vi "generateOriGrating.vi"(0 "Y resolution":i32=128, 1 "Square?":bool, 2 "New Image":T1, 5 "X resolution":i32, 7 "frequency (cyc/pixel)":dbl=0.0078125 format="%0.4e", 9 "Angle (degrees)":sgl format="%.2f", 11 "error in (no error)":errorcluster, 12 "phase in":dbl format="%0.2f") -> (4 "Image Dst Out":T1, 15 "error out":errorcluster)   [LabVIEW 2014]
uses:
  <vilib>/vision/Image Controls.llb/IMAQ Image.ctl
  <vilib>/Analysis/baseanly.llb/Real Outer Product.vi
  <vilib>/Analysis/Matrix/Numeric/Multiply/Multiply - RM,R.vi
  <vilib>/Analysis/NI_AALBase.lvlib
  <vilib>/Analysis/Matrix/NI_Matrix.lvlib
  <vilib>/vision/NI_Vision_Development_Module.lvlib
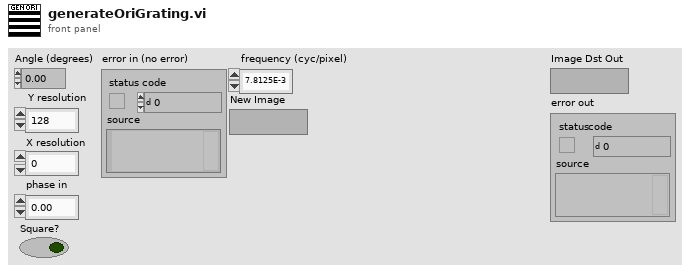
[diagram p1: front panel]
types:
  T1 = typedef "IMAQ Image.ctl" = refnum<image>
  T2 = typedef "NI_Matrix.lvlib/RealMatrix.ctl" = dbl[][]
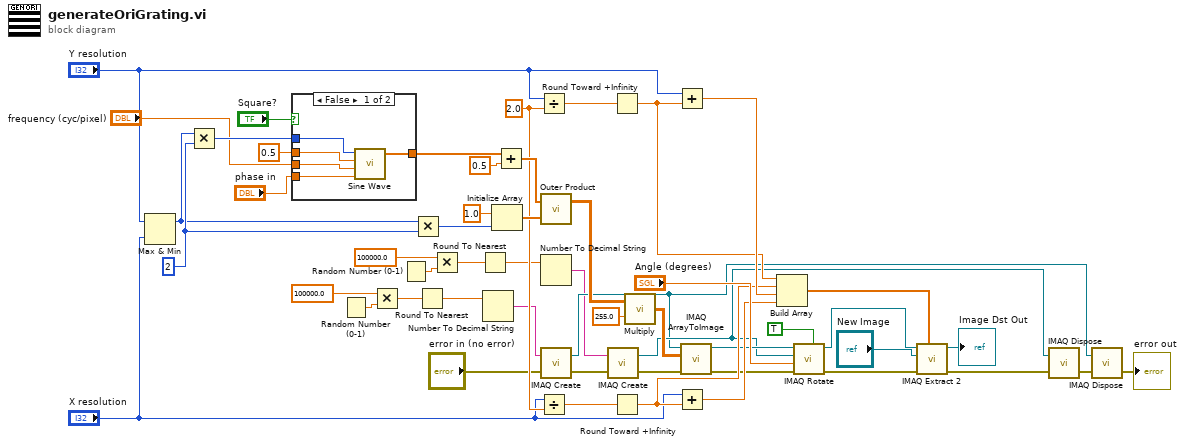
[diagram p0: block diagram]
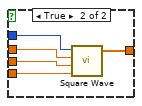
[diagram p2: hidden frame]
diagram:
  w36 = 2.0 ("y")
  w38 = 2
  n1 = Max & Min(x="Y resolution", y="X resolution") -> (max(x,y)=w1:i32)  [unwired: 1 out]
  n2 = Multiply(x=w1, y=w38) -> (x*y=w37:i32)
  n3 = case shown="False" "Square?" {
    tunnel: 0.5 ("amplitude") -> [w56 w62]
    tunnel: "frequency (cyc/pixel)" -> [w53 w61]
    tunnel: [w54 w60] -> w49
    tunnel: w37 -> [w57 w59]
    tunnel: "phase in" -> [w55 w58]
    frame False {
      n4 = call <vilib>:"Sine Wave.vi"("samples"=w57, "amplitude"=w56, "frequency"=w53, "phase in"=w55) -> ("sine wave"=w54:dbl[])  [unwired: 1 in, 2 out]
    }
    frame True {
      n5 = call <vilib>:"Square Wave.vi"("samples"=w59, "amplitude"=w62, "frequency"=w61, "phase in"=w58) -> ("square wave"=w60:dbl[])  [unwired: 2 in, 2 out]
    }
  }
  n6 = Random Number (0-1)() -> (number: 0 to 1=w13:dbl)
  n7 = Multiply(x=100000.0, y=w13) -> (x*y=w11:dbl)
  n8 = Random Number (0-1)() -> (number: 0 to 1=w5:dbl)
  n9 = Multiply(x=w1, y=w38) -> (x*y=w39:i32)
  n10 = Round To Nearest(number=w11) -> (nearest integer value=w10:dbl)
  n11 = Multiply(x=100000.0, y=w5) -> (x*y=w7:dbl)
  n12 = Round To Nearest(number=w7) -> (nearest integer value=w8:dbl)
  n13 = Number To Decimal String(number=w10) -> (decimal integer string=w9:string)  [unwired: 1 in]
  n14 = Initialize Array(1.0 ("element"), w39) -> (w51:dbl[])
  n15 = Add(x=w49, y=0.5) -> (x+y=w47:dbl[])
  n16 = Divide(x="Y resolution", y=w36) -> (x/y=w32:dbl)
  n17 = Divide(x="X resolution", y=w36) -> (x/y=w30:dbl)
  n18 = call-poly <vilib>:"Outer Product.vi"("Y Vector"=w51, "X Vector"=w47) -> ("Outer Product"=w45:T2)  [unwired: 1 out]
  n19 = Number To Decimal String(number=w8) -> (decimal integer string=w4:string)  [unwired: 1 in]
  n20 = call "IMAQ Create"("Image Name"=w9, "error in (no error)"="error in (no error)") -> ("New Image"=w14:T1, "error out"=w20:errorcluster)  [unwired: 3 in]
  n21 = call "IMAQ Create"("Image Name"=w4, "error in (no error)"=w20) -> ("New Image"=w15:T1, "error out"=w19:errorcluster)  [unwired: 3 in]
  n22 = Round Toward +Infinity(x=w32) -> (ceil(x): smallest int >= x=w31:dbl)
  n23 = Round Toward +Infinity(x=w30) -> (ceil(x): smallest int >= x=w29:dbl)
  n24 = call-poly <vilib>:"Multiply.vi"("Real Scalar c"=255.0 ("y"), "Real Matrix A"=w45) -> ("A * c"=w44:T2)
  n25 = Add(x="Y resolution", y=w31) -> (x+y=w34:dbl)
  n26 = Add(x="X resolution", y=w29) -> (x+y=w33:dbl)
  n27 = call "IMAQ ArrayToImage"("error in (no error)"=w19, "Image Pixels (U8)"=w44, "Image"=w14) -> ("error out"=w23:errorcluster, "Image Out"=w24:T1)  [unwired: 7 in]
  n28 = Build Array(w31, w29, w34, w33) -> (w35:dbl[])
  n29 = call "IMAQ Rotate"("Maintain Size"=TRUE, "error in (no error)"=w23, "Angle (degrees)"="Angle (degrees)", "Image Dst"=w15, "Image Src"=w24) -> ("error out"=w26:errorcluster, "Image Dst Out"=w25:T1)  [unwired: 5 in]
  n30 = call "IMAQ Extract 2"("Optional Rectangle"=w35, "error in (no error)"=w26, "Image Dst"="New Image", "Image Src"=w25) -> ("error out"=w18:errorcluster, "Image Dst Out"=→"Image Dst Out":T1)  [unwired: 6 in]
  n31 = call "IMAQ Dispose"("Image"=w15, "error in (no error)"=w18) -> ("error out"=w17:errorcluster)  [unwired: 4 in]
  n32 = call "IMAQ Dispose"("Image"=w14, "error in (no error)"=w17) -> ("error out"=→"error out":errorcluster)  [unwired: 4 in]
